vi "Replace First and Last Words in String.vi"(10 "sorted array":T1[](array[typedef]), 11 "String in":string) -> (3 "String out":string)   [LabVIEW 2020, in "Words to Numbers Converter.lvclass"]
uses:
  Words to Numbers Converter.lvclass
  Word in String.ctl
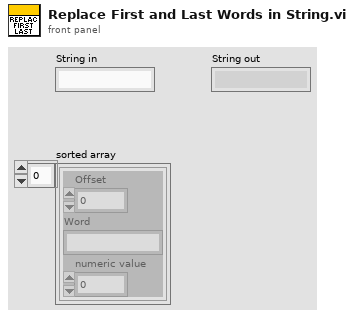
[diagram p1: front panel]
types:
  T1 = typedef "Words to Numbers Converter.lvclass/Word in String.ctl" = cluster{"Offset":i32, "Word":string, "numeric value":i32}
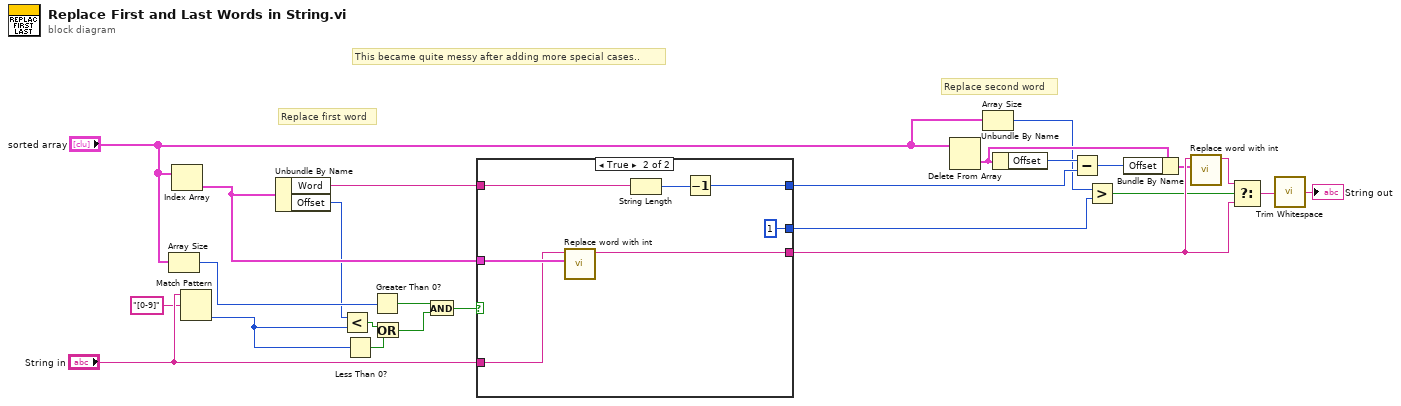
[diagram p0: block diagram]
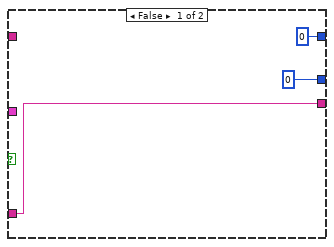
[diagram p2: hidden frame]
diagram:
  # "Replace second word"
  # "Replace first word"
  # "This became quite messy after adding more special cases.."
  n1 = Array Size(array="sorted array") -> (size(s)=w21:i32)
  n2 = Index Array(array="sorted array") -> (element=w16:T1)  [unwired: 1 in]
  n3 = Match Pattern(string="String in", regular expression="[0-9]") -> (offset past match=w7:i32)  [unwired: 1 in, 3 out]
  n4 = Unbundle By Name(w16) -> ("Word"=w19:string, "Offset"=w8:i32)
  n5 = Less?(x=w8, y=w7) -> (x < y?=w6:bool)
  n6 = Less Than 0?(x=w7) -> (x < 0?=w5:bool)
  n7 = Greater Than 0?(x=w21) -> (x > 0?=w22:bool)
  n8 = Or(x=w6, y=w5) -> (x .or. y?=w3:bool)
  n9 = And(x=w22, y=w3) -> (x .and. y?=w4:bool)
  n10 = case shown="True" w4 {
    tunnel: [w27 w31] -> w25
    tunnel: [0 w35] -> w20
    tunnel: w19 -> [_ w34]
    tunnel: w16 -> [_ w32]
    tunnel: "String in" -> [w27 w30]
    tunnel: [0 ("y") 1 ("y")] -> w2
    frame False {
    }
    frame True {
      n11 = call "Replace word with int.vi"("Cluster"=w32, "String in"=w30) -> ("String out"=w31:string)  [unwired: 9 in]
      n12 = String Length(string=w34) -> (length=w33:i32)
      n13 = Decrement(x=w33) -> (x-1=w35:i32)
    }
  }
  n14 = Delete From Array(array="sorted array") -> (deleted portion=w14:T1)  [unwired: 2 in, 1 out]
  n15 = Array Size(array="sorted array") -> (size(s)=w11:i32)
  n16 = Unbundle By Name(w14) -> ("Offset"=w17:i32)
  n17 = Subtract(x=w17, y=w20) -> (x-y=w18:i32)
  n18 = Greater?(x=w11, y=w2) -> (0:w24:bool)
  n19 = Bundle By Name(cluster=w14, "Offset"=w18) -> (w15:T1)
  n20 = call "Replace word with int.vi"("Cluster"=w15, "String in"=w25) -> ("String out"=w13:string)  [unwired: 9 in]
  n21 = Select(t=w13, s=w24, f=w25) -> (s? t:f=w23:string)
  n22 = call <vilib>:"Trim Whitespace.vi"("string"=w23) -> ("trimmed string"=→"String out":string)  [unwired: 1 in]
